vi "Test Adding Nested Test Cases.vi"(8 "error in (no error)":errorcluster, 11 "Result Model Tests in":refnum<class "Result Model Tests.lvclass">) -> (0 "error out":errorcluster, 3 "Result Model Tests out":refnum<class "Result Model Tests.lvclass">)   [LabVIEW 2020, in "Result Model Tests.lvclass"]
uses:
  Result Model Tests.lvclass
  Result Model Tests.lvclass/Result Model Tests.ctl
  Result Model/Result Model.lvclass
  206db1ee-aa99-40b9-8881-171f2a77c34b.vi
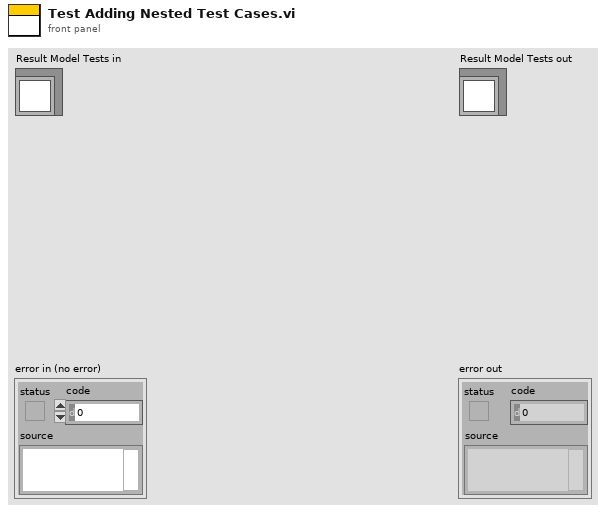
[diagram p1: front panel]
types:
  T1 = cluster{"Left Cell String":string, "Child Text":string[], "Child Tag":string, "Item Indent":i32, "Child Only?":bool, "Glyph Index":i32}[]
  T2 = cluster{"Left Cell String":string, "Child Text":string[], "Child Tag":string, "Item Indent":i32, "Child Only?":bool, "Glyph Index":i32}
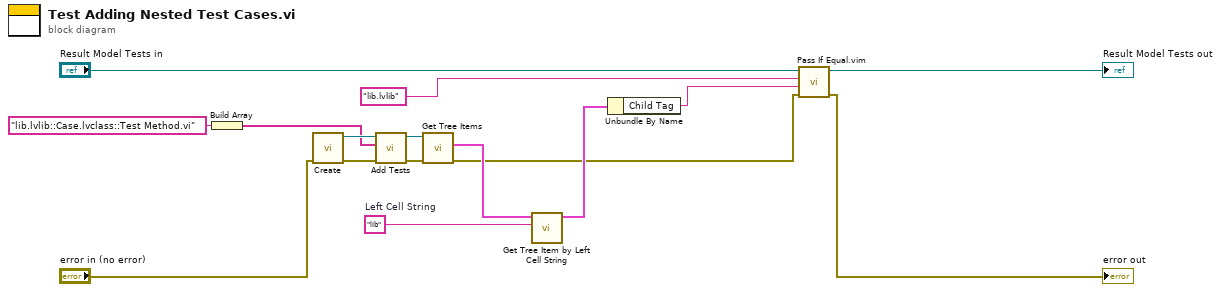
[diagram p0: block diagram]
diagram:
  w2 = "lib"  # Left Cell String
  n1 = Build Array("lib.lvlib::Case.lvclass::Test Method.vi" ("String")) -> (w6:string[])
  n2 = call "Create.vi"("error in (no error)"="error in (no error)") -> ("error out"=w14:errorcluster, "Result Model out"=w15:refnum<class "Result Model.lvclass">)  [unwired: 9 in]
  n3 = call "Add Tests.vi"("error in (no error)"=w14, "Tests"=w6, "Result Model In"=w15) -> ("error out"=w12:errorcluster, "Result Model Out"=w13:refnum<class "Result Model.lvclass">)  [unwired: 7 in]
  n4 = call "Get Tree Items.vi"("error in (no error)"=w12, "Result Model In"=w13) -> ("error out"=w4:errorcluster, "Tree Items"=w10:T1)  [unwired: 7 in, 1 out]
  n5 = call "Get Tree Item by Left Cell String.vi"("Left Cell String"=w2, "Tree Items"=w10) -> ("Item"=w8:T2)  [unwired: 9 in]
  n6 = Unbundle By Name(w8) -> ("Child Tag"=w7:string)
  n7 = call "Pass If Equal.vim"("error in (no error)"=w4, "Actual"=w7, "Expected"="lib.lvlib" ("String"), "LUnit Test Case In"="Result Model Tests in") -> ("error out"=→"error out":errorcluster, "LUnit Test Case Out"=→"Result Model Tests out":refnum<class "Result Model Tests.lvclass">)  [unwired: 6 in]
